vi "SaveTreeUISettings.vi"(8 "Error In":errorcluster, 11 "UI References":T1) -> (0 "Error Out":errorcluster)   [LabVIEW 2017, in "Client.lvlib" / "UI_API.lvlib"]
uses:
  UI_API.lvlib
  TypeDefs/UIReferences.ctl
  ClientGlobals.vi
  <vilib>/Utility/config.llb/Write Key (I32).vi
  <vilib>/Utility/config.llb/Write Key (String).vi
  <vilib>/Utility/config.llb/NI_LVConfig.lvlib
  Client.lvlib
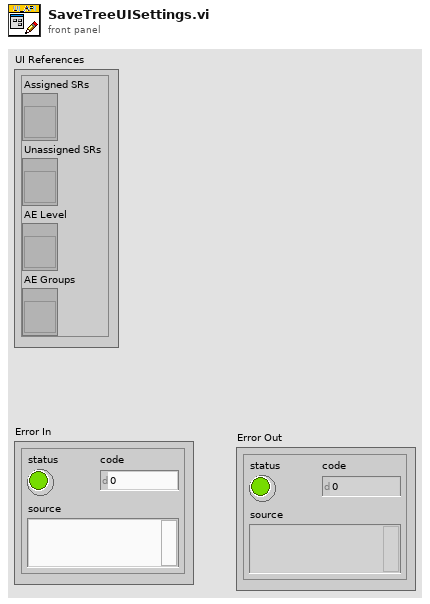
[diagram p1: front panel]
types:
  T1 = typedef "Client.lvlib/UI_API.lvlib/UIReferences.ctl" = cluster{"Assigned SRs":refnum<vi>, "Unassigned SRs":refnum<vi>, "AE Level":refnum<vi>, "AE Groups":refnum<vi>}
  T2 = typedef "NI_LVConfig.lvlib/Config Data RefNum.ctl" = refnum<k1>
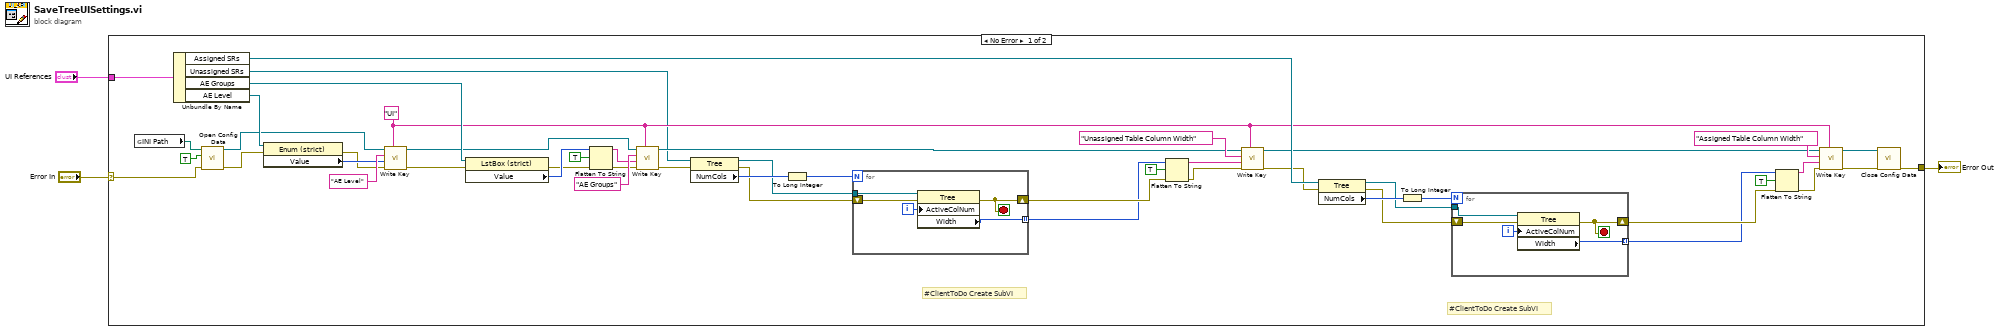
[diagram p0: block diagram]
diagram:
  n1 = case shown="No Error" "Error In" {
    selector: "Error In" -> [w51 w63]
    tunnel: "UI References" -> [w50 _]
    tunnel: [w34 w63] -> w1
    frame No Error {
      w19 = "UI" ("section")
      # "#ClientToDo Create SubVI"
      # "#ClientToDo Create SubVI"
      n2 = global read "ClientGlobals.vi" "INI Path"() -> (w18:path)
      n3 = Unbundle By Name(w50) -> ("Assigned SRs"=w28:refnum<vi>, "Unassigned SRs"=w16:refnum<vi>, "AE Groups"=w42:refnum<vi>, "AE Level"=w48:refnum<vi>)
      n4 = call <vilib>:"Open Config Data.vi"("error in (no error)"=w51, "create file if necessary (T)"=TRUE ("create file if necessary? (T)"), "configuration file path"=w18) -> ("error out"=w46:errorcluster, "refnum"=w44:T2)  [unwired: 6 in, 1 out]
      n5 = property class="Enum (strict)"(reference=w48, error in=w46) -> (error out=w45:errorcluster, "Value"=w47:enum16{"AE / ELP", "AE Intern"})  [unwired: 1 out]
      n6 = call-poly <vilib>:"Write Key.vi"("section"=w19, "error in (no error)"=w45, "value"=w47, "key"="AE Level", "refnum"=w44) -> ("error out"=w41:errorcluster, "refnum out"=w35:T2)  [unwired: 4 in, 1 out]
      n7 = property class="LstBox (strict)"(reference=w42, error in=w41) -> (error out=w37:errorcluster, "Value"=w40:i32[])  [unwired: 1 out]
      n8 = Flatten To String(anything=w40, prepend array or string size? (T)=TRUE, error in (no error)=w37) -> (data string=w38:string, error out=w36:errorcluster)  [unwired: 1 in, 1 out]
      n9 = call-poly <vilib>:"Write Key.vi"("section"=w19, "error in (no error)"=w36, "value"=w38, "key"="AE Groups", "refnum"=w35) -> ("error out"=w15:errorcluster, "refnum out"=w17:T2)  [unwired: 4 in, 1 out]
      n10 = property class="Tree"(reference=w16, error in=w15) -> (reference out=w11:refnum<vi>, error out=w13:errorcluster, "NumCols"=w14:u32)
      n11 = To Long Integer(number=w14) -> (32bit integer=w12:i32)
      n12 = for {
        N: w12 -> [_]
        shift-right: [w60] -> w10
        shift-left: w13 -> [w61]
        tunnel: w11 -> [w62]
        tunnel: [w58] -> w9 mode=indexing
        i -> [w59]
        stop <- w60 stop-if-true
        n13 = property class="Tree"(reference=w62, error in=w61, "ActiveColNum"=w59) -> (error out=w60:errorcluster, "Width"=w58:i32)  [unwired: 1 out]
      }
      n14 = Flatten To String(anything=w9, prepend array or string size? (T)=TRUE, error in (no error)=w10) -> (data string=w31:string, error out=w32:errorcluster)  [unwired: 1 in, 1 out]
      n15 = call-poly <vilib>:"Write Key.vi"("section"=w19, "error in (no error)"=w32, "value"=w31, "key"="Unassigned Table Column Width", "refnum"=w17) -> ("error out"=w26:errorcluster, "refnum out"=w24:T2)  [unwired: 4 in, 1 out]
      n16 = property class="Tree"(reference=w28, error in=w26) -> (reference out=w4:refnum<vi>, error out=w8:errorcluster, "NumCols"=w29:u32)
      n17 = To Long Integer(number=w29) -> (32bit integer=w6:i32)
      n18 = for {
        N: w6 -> [_]
        shift-right: [w56] -> w7
        shift-left: w8 -> [w57]
        tunnel: [w54] -> w5 mode=indexing
        tunnel: w4 -> [w53]
        i -> [w55]
        stop <- w56 stop-if-true
        n19 = property class="Tree"(reference=w53, error in=w57, "ActiveColNum"=w55) -> (error out=w56:errorcluster, "Width"=w54:i32)  [unwired: 1 out]
      }
      n20 = Flatten To String(anything=w5, prepend array or string size? (T)=TRUE, error in (no error)=w7) -> (data string=w20:string, error out=w21:errorcluster)  [unwired: 1 in, 1 out]
      n21 = call-poly <vilib>:"Write Key.vi"("section"=w19, "error in (no error)"=w21, "value"=w20, "key"="Assigned Table Column Width", "refnum"=w24) -> ("error out"=w25:errorcluster, "refnum out"=w23:T2)  [unwired: 4 in, 1 out]
      n22 = call <vilib>:"Close Config Data.vi"("error in (no error)"=w25, "refnum"=w23) -> ("error out"=w34:errorcluster)  [unwired: 8 in, 1 out]
    }
    frame Error {
    }
  }
  "Error Out" <- w1
